vi "save_to_db.vi"(3 "error in":errorcluster, 5 "Raw Signal 3":waveform(dbl)[](array[waveform])) -> (0 "error out":errorcluster)   [LabVIEW 2018]
uses:
  <vilib>/drjdpowell/SQLite Library/SQL Statement/SQL Statement.lvclass/SQL Statement.ctl
  <vilib>/drjdpowell/SQLite Library/SQL Connection/Open (path).vi
  <vilib>/drjdpowell/SQLite Library/SQL Statement/Bind Real.vi
  <vilib>/drjdpowell/SQLite Library/SQL Statement/Bind Timestamp (Text).vi
  <vilib>/drjdpowell/SQLite Library/SQL Connection/Open (string).vi
  <vilib>/drjdpowell/SQLite Library/SQL Statement/Step.vi
  <vilib>/JDP Science/JDP Science Common Utilities/Timestamp/Timestamp to Text.vi
  <vilib>/drjdpowell/SQLite Library/SQL Statement/Bind UTF-8 Text.vi
  <vilib>/AdvancedString/Path To Command Line String.vi
  <vilib>/drjdpowell/SQLite Library/SQL Statement/Error Message.vi
  <vilib>/drjdpowell/SQLite Library/SQL Connection/Connection.lvclass
  <vilib>/drjdpowell/SQLite Library/SQL Statement/SQL Statement.lvclass
  <vilib>/drjdpowell/SQLite Library/Transaction Helpers/Transaction.lvlib
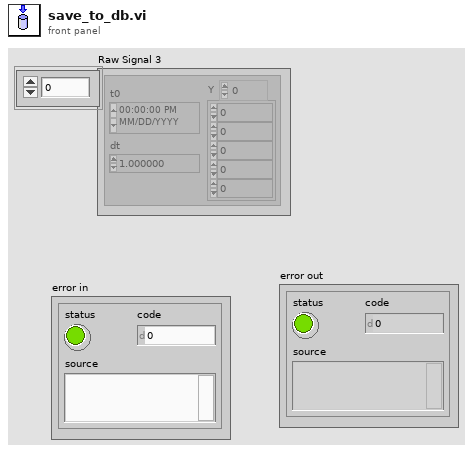
[diagram p1: front panel]
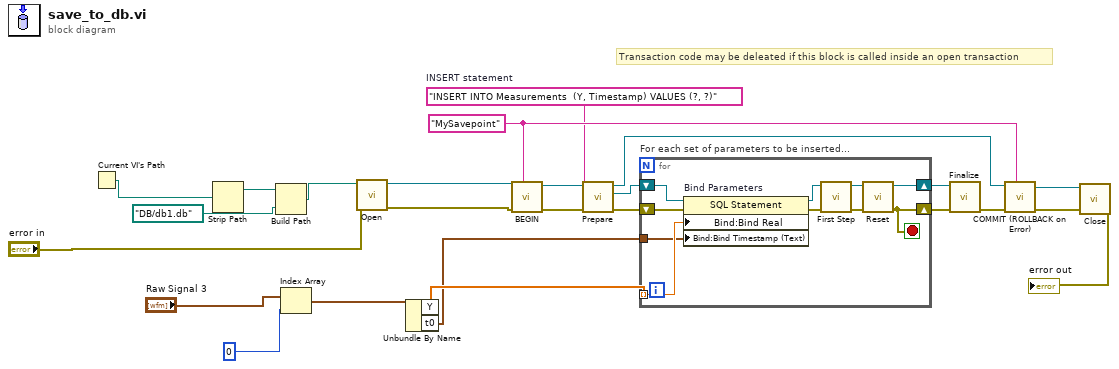
[diagram p0: block diagram]
diagram:
  w19 = "MySavepoint" ("Savepoint name")
  w14 = "INSERT INTO Measurements  (Y, Timestamp) VALUES (?, ?)"  # INSERT statement
  # "Transaction code may be deleated if this block is called inside an open transaction"
  n1 = Current VI's Path() -> (path=w25:path)
  n2 = Strip Path(path=w25) -> (stripped path=w24:path)  [unwired: 1 out]
  n3 = Build Path(base path=w24, name or relative path=path "DB/db1.db") -> (appended path=w23:path)
  n4 = Index Array(array="Raw Signal 3", index=0) -> (element=w7:waveform(dbl))
  n5 = call-poly <vilib>:"Open.vi"("error in (no error)"="error in", "db file"=w23) -> ("error out"=w4:errorcluster, "SQLite Connection"=w11:refnum<class "Connection.lvclass">)  [unwired: 8 in]
  n6 = Unbundle By Name(w7) -> ("Y"=w6:dbl[], "t0"=w1:timestamp)
  n7 = call <vilib>:"BEGIN.vi"("Savepoint name"=w19, "error in (no error)"=w4, "SQLite Connection in"=w11) -> ("error out"=w18:errorcluster, "SQLite Connection"=w17:refnum<class "Connection.lvclass">)  [unwired: 7 in]
  n8 = call <vilib>:"Prepare.vi"("error in (no error)"=w18, "SQL"=w14, "SQLite Connection in"=w17) -> ("error out"=w13:errorcluster, "SQL Statement"=w12:refnum<class "SQL Statement.lvclass">, "SQLite Connection"=w20:refnum<class "Connection.lvclass">)  [unwired: 4 in, 2 out]
  n9 = for "For each set of parameters to be inserted..." {
    shift-right: [w29] -> w15
    shift-left: w12 -> [w35]
    shift-right: [w28] -> w16
    shift-left: w13 -> [w32]
    tunnel: w6 -> [w27] mode=indexing
    tunnel: w1 -> [w26]
    stop <- w28 stop-if-true
    n10 = property on="Bind Parameters" class="SQL Statement"(reference=w35, error in=w32, "Bind:Bind Real"=w27, "Bind:Bind Timestamp (Text)"=w26) -> (reference out=w34:refnum<class "SQL Statement.lvclass">, error out=w33:errorcluster)
    n11 = call <vilib>:"First Step.vi"("error in (no error)"=w33, "SQL Statement in"=w34) -> ("error out"=w31:errorcluster, "SQL Statement"=w30:refnum<class "SQL Statement.lvclass">)  [unwired: 7 in, 1 out]
    n12 = call <vilib>:"Reset.vi"("error in (no error)"=w31, "SQL Statement in"=w30) -> ("error out"=w28:errorcluster, "SQL Statement"=w29:refnum<class "SQL Statement.lvclass">)  [unwired: 8 in]
  }
  n13 = call <vilib>:"Finalize.vi"("error in (no error)"=w16, "SQL Statement in"=w15) -> ("error out"=w21:errorcluster)  [unwired: 9 in]
  n14 = call <vilib>:"COMMIT (ROLLBACK on Error).vi"("Savepoint name"=w19, "error in (no error)"=w21, "SQLite Connection in"=w20) -> ("error out"=w3:errorcluster, "SQLite Connection"=w10:refnum<class "Connection.lvclass">)  [unwired: 7 in]
  n15 = call-dynamic "Close.vi"("error in (no error)"=w3, "SQLite Connection in"=w10) -> ("error out"=→"error out":errorcluster)  [unwired: 9 in]
